vi "Write Save_.vi"(8 "error in (no error)":errorcluster, 10 "Save?":bool, 11 "Save Data MSG in":refnum<class "Save Data MSG.lvclass">) -> (0 "error out":errorcluster, 3 "Save Data MSG out":refnum<class "Save Data MSG.lvclass">)   [LabVIEW 2014, in "Controller.lvlib" / "Save Data MSG.lvclass"]
uses:
  Save Data MSG.lvclass
  Save Data MSG.lvclass/Save Data MSG.ctl
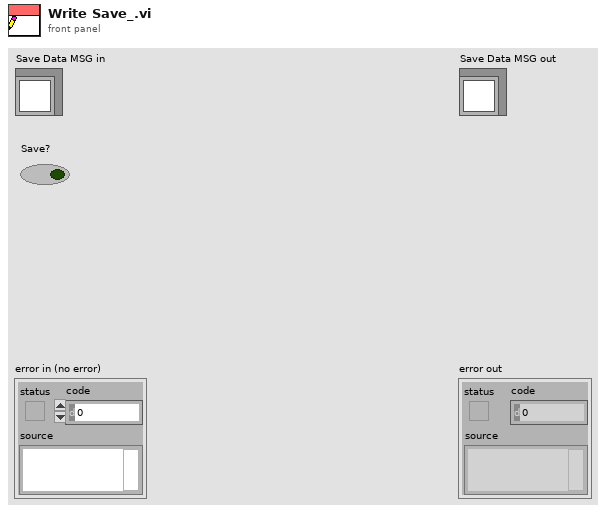
[diagram p1: front panel]
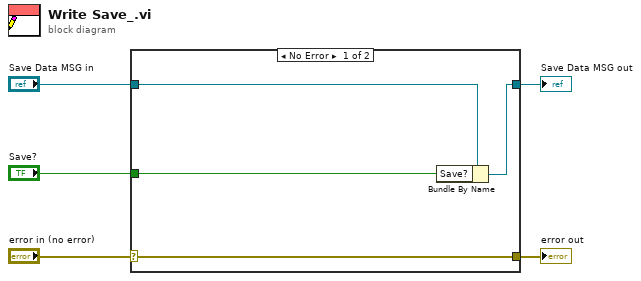
[diagram p0: block diagram]
diagram:
  n1 = case shown="No Error" "error in (no error)" {
    selector: "error in (no error)" -> [w9 w10]
    tunnel: [w9 w10] -> w4
    tunnel: [w7 w11] -> w2
    tunnel: "Save Data MSG in" -> [w8 w11]
    tunnel: "Save?" -> [w6 _]
    frame No Error {
      n2 = Bundle By Name(cluster=w8, "Save?"=w6) -> (w7:refnum<class "Save Data MSG.lvclass">)
    }
    frame Error {
    }
  }
  "error out" <- w4
  "Save Data MSG out" <- w2
